vi "Init Events.vi"(8 "error in (no error)":errorcluster, 11 "DAQ_Engine in":refnum<class "DAQ_Engine.lvclass">) -> (0 "error out":errorcluster, 3 "DAQ_Engine out":refnum<class "DAQ_Engine.lvclass">)   [LabVIEW 2019, in "DAQ_Engine.lvclass"]
doc: "Developed by Kevin Thompson\nkevin@thompsonengineering.net\n\nCopyright 2018\nThompson Engineering, LLC"
uses:
  DAQ_Engine.lvclass
  Common/DataTypes/TD Async CmdMsg EventData--cluster.ctl
  DataTypes/DAQStateChg EvData--cluster.ctl
  DataTypes/DAQStateEvData--cluster.ctl
  Common/DataTypes/DAQState--enum.ctl
  DataTypes/DAQMeasSettingsChg EvData--cluster.ctl
  DataTypes/DAQMeasSettingsEvData--cluster.ctl
  Common/DataTypes/Measurement Config--cluster.ctl
  DataTypes/DAQAcqModeChg EvData--cluster.ctl
  Common/DataTypes/Acquisition Mode--cluster.ctl
  DAQ_Engine.lvclass/DAQ_Engine.ctl
  Accessors/Get PublicEvents.vi
  Accessors/Set PublicEvents.vi
  Accessors/Get ObjData.vi
  Accessors/Set ObjData.vi
  Config/Config.lvclass
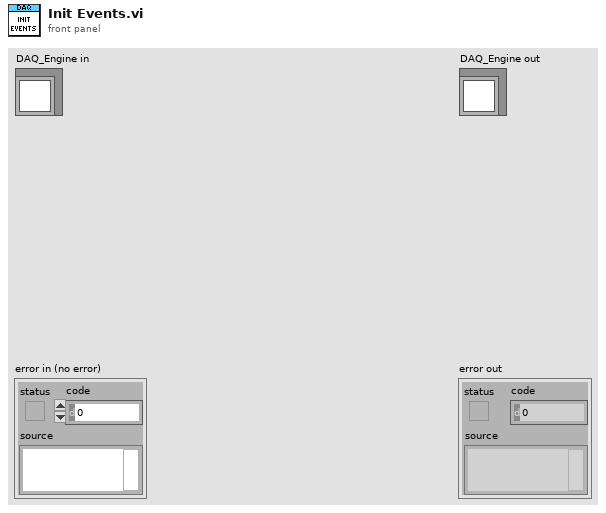
[diagram p1: front panel]
types:
  T1 = typedef "DAQ_Engine.lvclass/DAQAcqModeChg EvData--cluster.ctl" = cluster{"Time Stamp":timestamp, "OLD AcqMode":T2, "NEW AcqMode":T2}
  T2 = typedef "Acquisition Mode--cluster.ctl" = enum16{"3phase", "Single"}
  T3 = typedef "DAQ_Engine.lvclass/DAQMeasSettingsChg EvData--cluster.ctl" = cluster{"Time Stamp":timestamp, "OLD Settings":T4, "NEW Settings":T4}
  T4 = typedef "DAQ_Engine.lvclass/DAQMeasSettingsEvData--cluster.ctl" = cluster{"Measurement config":T5, "vData":variant}
  T5 = typedef "Measurement Config--cluster.ctl" = cluster{"Data Rate 9775":dbl, "Data Rate 9215":dbl, "Samples RMS 9215":u32, "Samples RMS 9775":u32}
  T6 = typedef "DAQ_Engine.lvclass/DAQStateChg EvData--cluster.ctl" = cluster{"Time Stamp":timestamp, "OLD State":T7, "NEW State":T7}
  T7 = typedef "DAQ_Engine.lvclass/DAQStateEvData--cluster.ctl" = cluster{"DAQState":T8, "vData":variant}
  T8 = typedef "DAQState--enum.ctl" = enum16{"Unknown", "Stopped", "Running", "Error"}
  T9 = typedef "TD Async CmdMsg EventData--cluster.ctl" = cluster{"Time Stamp":timestamp, "CmdMsg":string, "vData":variant}
  T10 = typedef "DAQ_Engine.lvclass/Public Events--cluster.ctl" = cluster{"DAQ_Engine.AsyncCmd Event":refnum<user-event>, "DAQ_Engine.AsyncMsg Event":refnum<user-event>, "stop process":refnum<user-event>, "DAQ_Engine.DAQStateChg Ev":refnum<user-event>, "DAQ_Engine.MeasSettingsChg Ev":refnum<user-event>, "DAQ_Engine.AcqModeChg Ev":refnum<user-event>}
  T11 = typedef "DAQ_Engine.lvclass/ObjData--cluster.ctl" = cluster{"Settings":T12, "Public Events":T10, "Dependency":T14, "ReadData-placeholder":T15, "VISA-placeholder":refnum<visa-resource-name>, "MeasSettings":T5, "InverterDataAcqMode":T2, "RawDaqDataQ":T16, "Private Events":T17, "DAQState Data":T7}
  T12 = typedef "DAQ_Engine.lvclass/Settings--cluster.ctl" = cluster{"Simulation":bool, "Initial ErrReporting setting":i32, "Initial Measurement settings":T5, "BoardNum":T13, "Acquisition mode":T2, "DemoMode":bool}
  T13 = typedef "DAQ_Engine.lvclass/BoardNum--cluster.ctl" = cluster{"P1Sgl":u32, "P2":u32, "P3":u32}
  T14 = typedef "DAQ_Engine.lvclass/Dependency--cluster.ctl" = cluster{"Config":refnum<class "Config.lvclass">}
  T15 = typedef "DAQ_Engine.lvclass/Read Data--cluster.ctl" = cluster{"Data":dbl}
  T16 = typedef "RawDAQDataQRef--cluster.ctl" = refnum<queue>
  T17 = typedef "DAQ_Engine.lvclass/Private Events--cluster.ctl" = cluster{"PrivateAsync Ev":refnum<user-event>}
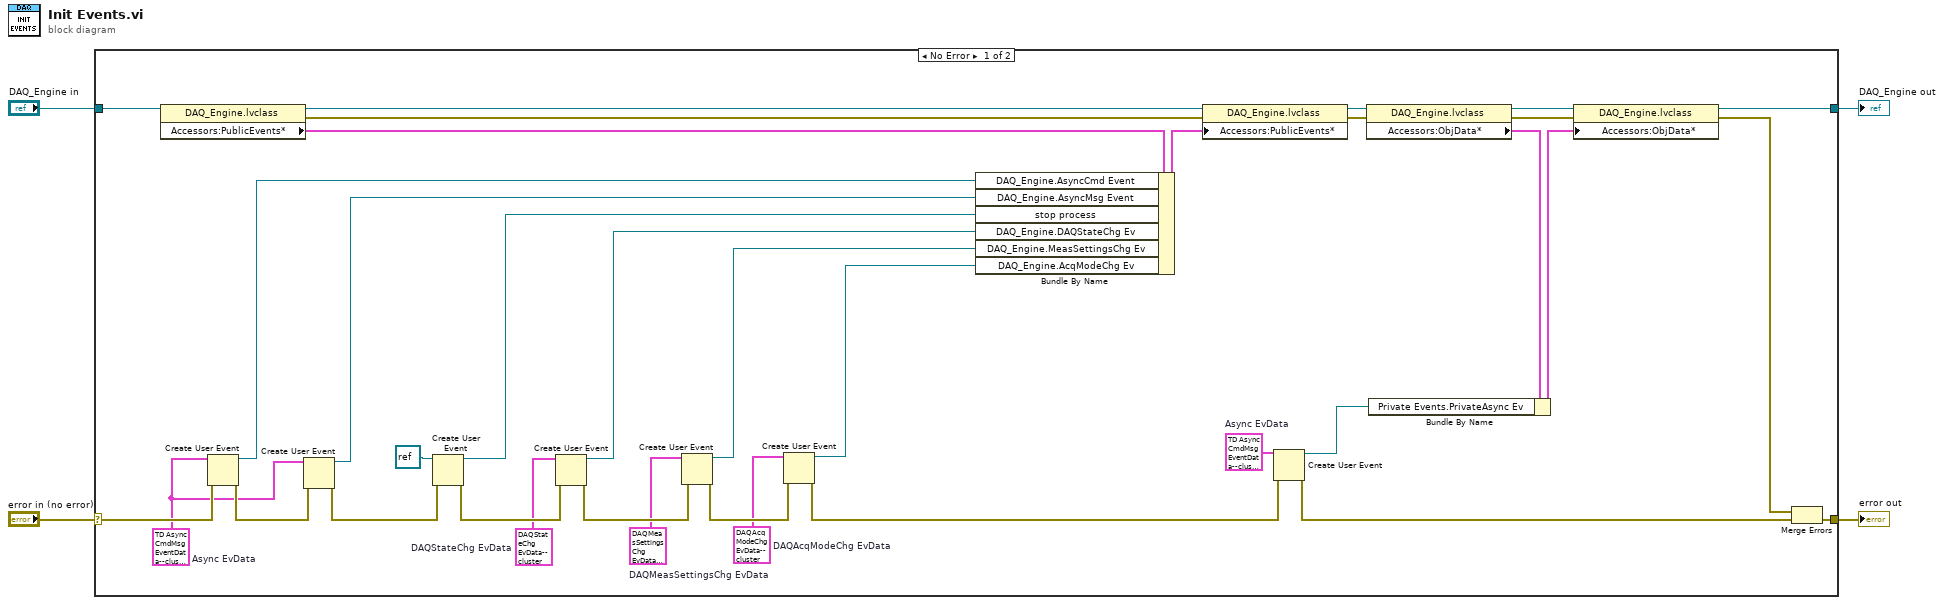
[diagram p0: block diagram]
diagram:
  n1 = case shown="No Error" "error in (no error)" {
    selector: "error in (no error)" -> [w31 w41]
    tunnel: [w7 w41] -> w3
    tunnel: [w12 w40] -> w1
    tunnel: "DAQ_Engine in" -> [w38 w40]
    frame No Error {
      w15 = T1 {"Time Stamp"=timestamp(0 s since 1904-01-01), "OLD AcqMode"=enum."3phase", "NEW AcqMode"=enum."3phase"}  # DAQAcqModeChg EvData
      w17 = T3 {"Time Stamp"=timestamp(0 s since 1904-01-01), "OLD Settings"={"Measurement config"={"Data Rate 9775"=3.0, "Data Rate 9215"=1200000.0, "Samples RMS 9215"=480000, "Samples RMS 9775"=3}, "vData"=variant}, "NEW Settings"={"Measurement config"={"Data Rate 9775"=3.0, "Data Rate 9215"=1200000.0, "Samples RMS 9215"=480000, "Samples RMS 9775"=3}, "vData"=variant}}  # DAQMeasSettingsChg EvData
      w22 = T6 {"Time Stamp"=timestamp(0 s since 1904-01-01), "OLD State"={"DAQState"=enum."Unknown", "vData"=variant}, "NEW State"={"DAQState"=enum."Unknown", "vData"=variant}}  # DAQStateChg EvData
      w26 = T9 {"Time Stamp"=timestamp(0 s since 1904-01-01), "CmdMsg"="", "vData"=variant}  # Async EvData
      w28 = T9 {"Time Stamp"=timestamp(0 s since 1904-01-01), "CmdMsg"="", "vData"=variant}  # Async EvData
      n2 = property class="DAQ_Engine.lvclass"(reference=w38) -> (reference out=w37:refnum<class "DAQ_Engine.lvclass">, error out=w5:errorcluster, "Accessors:PublicEvents*"=w36:T10)  [unwired: 1 in]
      n3 = Create User Event(user event datatype=w28, error in=w31) -> (user event=w32:refnum<user-event>, error out=w30:errorcluster)
      n4 = Create User Event(user event datatype=w28, error in=w30) -> (user event=w27:refnum<user-event>, error out=w29:errorcluster)
      n5 = Create User Event(user event datatype=refnum<notifier> refnum ("notifier out"), error in=w29) -> (user event=w33:refnum<user-event>, error out=w23:errorcluster)
      n6 = Create User Event(user event datatype=w22, error in=w23) -> (user event=w21:refnum<user-event>, error out=w20:errorcluster)
      n7 = Create User Event(user event datatype=w17, error in=w20) -> (user event=w16:refnum<user-event>, error out=w19:errorcluster)
      n8 = Create User Event(user event datatype=w15, error in=w19) -> (user event=w14:refnum<user-event>, error out=w18:errorcluster)
      n9 = Bundle By Name(cluster=w36, "DAQ_Engine.AsyncCmd Event"=w32, "DAQ_Engine.AsyncMsg Event"=w27, "stop process"=w33, "DAQ_Engine.DAQStateChg Ev"=w21, "DAQ_Engine.MeasSettingsChg Ev"=w16, "DAQ_Engine.AcqModeChg Ev"=w14) -> (w35:T10)
      n10 = property class="DAQ_Engine.lvclass"(reference=w37, error in=w5, "Accessors:PublicEvents*"=w35) -> (reference out=w39:refnum<class "DAQ_Engine.lvclass">, error out=w9:errorcluster)
      n11 = Create User Event(user event datatype=w26, error in=w18) -> (user event=w24:refnum<user-event>, error out=w25:errorcluster)
      n12 = property class="DAQ_Engine.lvclass"(reference=w39, error in=w9) -> (reference out=w13:refnum<class "DAQ_Engine.lvclass">, error out=w8:errorcluster, "Accessors:ObjData*"=w11:T11)
      n13 = Bundle By Name(cluster=w11, "Private Events.PrivateAsync Ev"=w24) -> (w10:T11)
      n14 = property class="DAQ_Engine.lvclass"(reference=w13, error in=w8, "Accessors:ObjData*"=w10) -> (reference out=w12:refnum<class "DAQ_Engine.lvclass">, error out=w6:errorcluster)
      n15 = Merge Errors(w6, w25) -> (w7:errorcluster)
    }
    frame Error {
    }
  }
  "error out" <- w3
  "DAQ_Engine out" <- w1
